vi "Main-Get and Set Height.vi"() -> ()   [LabVIEW 2014]
uses:
  Main-Stage-Based/(Global) Current handle and LaserPower_YCC.vi
  <vilib>/DAQmx/create/channels.llb/DAQmx Create Channel (AI-Voltage-Basic).vi
  <vilib>/DAQmx/configure/timing.llb/DAQmx Timing (Sample Clock).vi
  <vilib>/DAQmx/read.llb/DAQmx Read (Analog 1D DBL 1Chan NSamp).vi
panel:
  out "Surface position (um)":dbl
  out "Stage Array Shift (nm)":dbl
  in  "Change power?":bool
  in  "Set power (mV)":dbl=1000.0
  in  "Filter type 2":T1(ring)=enum."Moving-window avg"
  out "step size (nm)":dbl
  out "inital Laser power":dbl
  out "Avg to Hz":dbl
  out "Expect - Real move (nm)\nStage Offset\n+=more move\n-=less move":dbl
  in  "Tab Control":enum32{"Raw QPDz-Stage", "Filtered QPDz-Stage"}(tab)
  out "Raw XY Graph":T2(graph)
  out "Filtered XY Graph":T2(graph)
  in  "Set Height":bool
  in  "Set Height (nm)":dbl=300.0
  out "True rate?":bool
  in  "Avg points":i32=500
  out "traveling time (s)":dbl
  in  "Sampling Rate":dbl=32000.0 format="%0.2f"
  out "Position after move up":dbl
  in  "1/2 range  (um)":dbl=0.7000000000000001 format="%.3f"
  in  "scan rate  (um/s)":dbl=0.7 format="%.3f"
  out "Real Current Commanded position (um)":dbl=48.46734101118563 format="%0.5f"
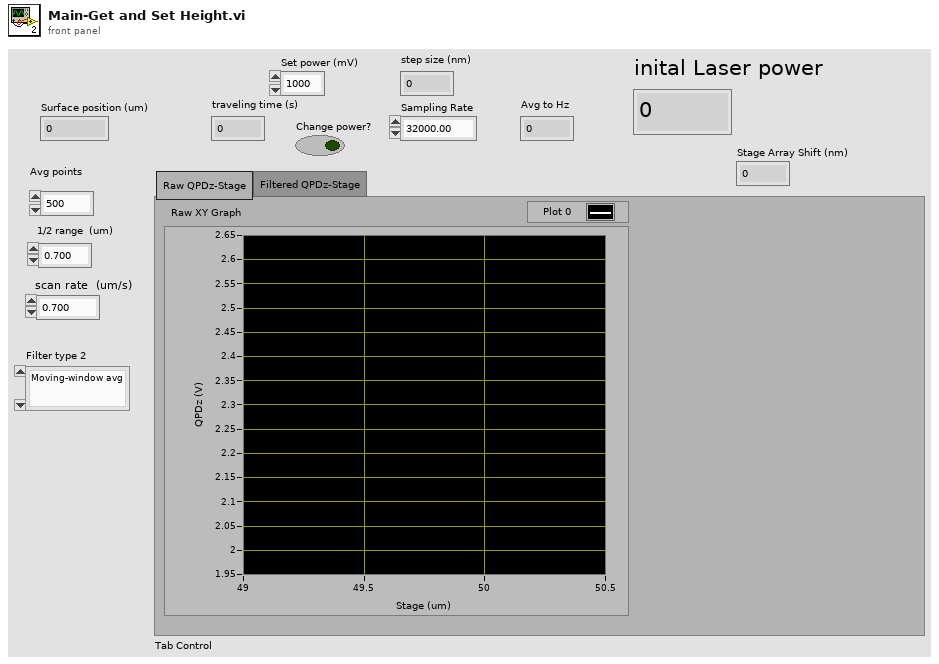
[diagram p1: front panel]
types:
  T1 = enum16{"Fixed-window avg", "Moving-window avg", "F+S-window avg", "S-G filter", "Fixed-window Median", "Moving-window Median "}
  T2 = cluster{"Filtered Stage Array":dbl[], "Filtered QPD data":dbl[]}
  T3 = cluster{"Correct Unfolded Stage Array (um)":dbl[], "Filtered QPD data":dbl[]}
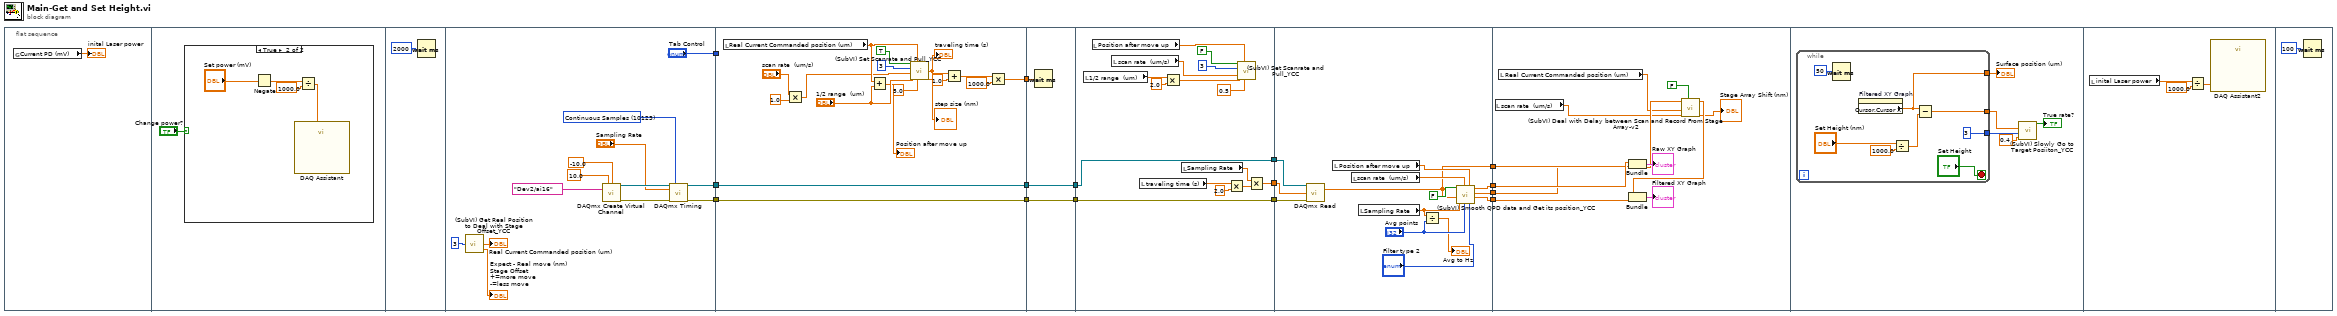
[diagram p0: block diagram]
diagram:
  n1 = flat-sequence {
    tunnel: [w26] -> w13
    tunnel: [w25] -> w9
    tunnel: ["Tab Control"] -> w1
    tunnel: [w46] -> w15
    tunnel: [w42] -> w14
    tunnel: w13 -> [w42]
    tunnel: [w41] -> w10
    tunnel: w9 -> [w41]
    tunnel: w1 -> [_]
    tunnel: w15 -> [w55]
    tunnel: w14 -> [w53]
    tunnel: [w54] -> w11
    tunnel: w10 -> [w54]
    tunnel: [w53] -> w7
    tunnel: [w66] -> w12
    tunnel: w11 -> [w66]
    tunnel: [w65] -> w8
    tunnel: w7 -> [w65]
    tunnel: [w63] -> w6
    tunnel: w12 -> [w84]
    tunnel: w8 -> [w83]
    tunnel: w6 -> [w82]
    tunnel: [w78] -> w5
    tunnel: [w77] -> w4
    tunnel: [w76] -> w3
    tunnel: [w75] -> w2
    tunnel: w5 -> [w90]
    tunnel: w4 -> [w95]
    tunnel: w3 -> [w94]
    tunnel: w2 -> [w93]
    frame #0 {
      n2 = global read "(Global) Current handle and LaserPower_YCC.vi" "Current PD (mV)"() -> (→"inital Laser power":dbl)
    }
    frame #1 {
      n3 = case shown="True" "Change power?" {
        frame False {
        }
        frame True {
          n4 = Negate(x="Set power (mV)") -> (-x=w20:dbl)
          n5 = Divide(x=w20, y=1000.0) -> (x/y=w18:dbl)
          n6 = call "DAQ Assistant"("data"=w18) -> ()  [unwired: 17 in, 2 out]
        }
      }
    }
    frame #2 {
      n7 = Wait (ms)(milliseconds to wait=u32 2000) -> ()  [unwired: 1 out]
    }
    frame #3 {
      w28 = 10123 items=["Finite Samples"=10178, "Continuous Samples"=10123, "Hardware Timed Single Point"=12522] ("sample mode")
      n8 = call "(SubVI) Get Real Position to Deal with Stage Offset_YCC.vi"("Axis"=3) -> ("Expect - Real move (nm)\nStage Offset\n+=more move\n-=less move"=→"Expect - Real move (nm)\nStage Offset\n+=more move\n-=less move":dbl, "Real Current Commanded position (um)"=→"Real Current Commanded position (um)":dbl)  [unwired: 3 in]
      n9 = call-poly <vilib>:"DAQmx Create Virtual Channel.vi"("maximum value"=10.0, "minimum value"=-10.0, "physical channels"=tag "Dev2/ai16") -> ("task out"=w29:refnum<k21>, "error out"=w30:errorcluster)  [unwired: 11 in]
      n10 = call-poly <vilib>:"DAQmx Timing.vi"("task/channels in"=w29, "sample mode"=w28, "rate"="Sampling Rate", "error in"=w30) -> ("task out"=w26:refnum<k21>, "error out"=w25:errorcluster)  [unwired: 10 in]
    }
    frame #4 {
      n11 = local read "Real Current Commanded position (um)"() -> (w45:dbl)
      n12 = Multiply(x="scan rate  (um/s)", y=1.0) -> (x*y=w36:dbl)
      n13 = Add(x=w45, y="1/2 range  (um)") -> (x+y=→"Position after move up":dbl)
      n14 = call "(SubVI) Set Scanrate and Pull_YCC.vi"("toward+ ?\nT=+, F=-"=TRUE ("toward+ ?\nT=+, F=-"), "Start From  (um)"=w45, "axis"=u32 3, "scan rate  (um/s)"=w36, "waiting time per point (ms)\nrange from 5ms to 0.167 ms"=5.0 ("waiting time per point (ms)\nrange from 5ms to 0.167 ms"), "range  (um)"="1/2 range  (um)") -> ("traveling time (s)"=w40:dbl, "step size (nm)"=→"step size (nm)":dbl)  [unwired: 1 out]
      "traveling time (s)" <- w40
      n15 = Add(x=w40, y=1.0) -> (x+y=w48:dbl)
      n16 = Multiply(x=w48, y=1000.0) -> (x*y=w46:dbl)
    }
    frame #5 {
      n17 = Wait (ms)(milliseconds to wait=w55) -> ()  [unwired: 1 out]
    }
    frame #6 {
      n18 = local read "1/2 range  (um)"() -> (w61:dbl)
      n19 = local read "Position after move up"() -> (w62:dbl)
      n20 = local read "scan rate  (um/s)"() -> (w68:dbl)
      n21 = local read "traveling time (s)"() -> (w57:dbl)
      n22 = Multiply(x=w61, y=2.0) -> (x*y=w59:dbl)
      n23 = local read "Sampling Rate"() -> (w64:dbl)
      n24 = Multiply(x=w57, y=2.0) -> (x*y=w56:dbl)
      n25 = call "(SubVI) Set Scanrate and Pull_YCC.vi"("toward+ ?\nT=+, F=-"=FALSE ("toward+ ?\nT=+, F=-"), "Start From  (um)"=w62, "axis"=u32 3, "scan rate  (um/s)"=w68, "waiting time per point (ms)\nrange from 5ms to 0.167 ms"=0.5 ("waiting time per point (ms)\nrange from 5ms to 0.167 ms"), "range  (um)"=w59) -> ()  [unwired: 3 out]
      n26 = Multiply(x=w64, y=w56) -> (x*y=w63:dbl)
    }
    frame #7 {
      n27 = call-poly <vilib>:"DAQmx Read.vi"("task/channels in"=w83, "number of samples per channel"=w82, "error in"=w84) -> ("data"=w75:dbl[])  [unwired: 10 in, 2 out]
      n28 = local read "Position after move up"() -> (w81:dbl)
      n29 = local read "scan rate  (um/s)"() -> (w80:dbl)
      n30 = local read "Sampling Rate"() -> (w74:dbl)
      n31 = Divide(x=w74, y="Avg points") -> (x/y=→"Avg to Hz":dbl)
      n32 = call "(SubVI) Smooth QPD data and Get its position_YCC.vi"("Filter type"="Filter type 2", "Initial position (um)"=w81, "Avg points"="Avg points", "scan rate  (um/s)"=w80, "Sampling rate (Hz)"=w74, "QPD data"=w75, "Direction\nT=+ \nF=-"=FALSE ("T=+ first\nF=- first")) -> ("Filtered QPD data"=w77:dbl[], "Filtered Stage Array"=w78:dbl[], "Raw Stage Array"=w76:dbl[])  [unwired: 2 in]
    }
    frame #8 {
      n33 = local read "scan rate  (um/s)"() -> (w87:dbl)
      n34 = local read "Real Current Commanded position (um)"() -> (w88:dbl)
      n35 = Bundle("Raw Stage Array"=w94, "data"=w93) -> (→"Raw XY Graph":cluster{"Raw Stage Array":dbl[], "data":dbl[]})  [unwired: 1 in]
      n36 = call "(SubVI) Deal with Delay between Scan and Record From Stage Array-v2.vi"("Toward first ?\nT=+, F=-"=FALSE ("Toward first ?\nT=+, F=-"), "Record scan rate  (um/s)"=w87, "Real initial position (um)"=w88, "Unfolded Stage Array (um)"=w90) -> ("Stage Array Shift (nm)"=→"Stage Array Shift (nm)":dbl, "Correct Unfolded Stage Array (um)"=w86:dbl[])  [unwired: 3 in, 1 out]
      n37 = Bundle("Correct Unfolded Stage Array (um)"=w86, "Filtered QPD data"=w95) -> (→"Filtered XY Graph":T3)  [unwired: 1 in]
    }
    frame #9 {
      n38 = while {
        tunnel: [w102] -> w99
        tunnel: [u32 3 ("axis")] -> w100
        tunnel: [w101] -> w96
        stop <- "Set Height" stop-if-true
        n39 = Wait (ms)(milliseconds to wait=u32 50) -> ()  [unwired: 1 out]
        n40 = property on="Filtered XY Graph" class="XYGraph (strict)"() -> ("Cursor.Cursor X"=w101:dbl)  [unwired: 2 in, 2 out]
        n41 = Divide(x="Set Height (nm)", y=1000.0) -> (x/y=w103:dbl)
        n42 = Subtract(x=w101, y=w103) -> (x-y=w102:dbl)
      }
      "Surface position (um)" <- w96
      n43 = call "(SubVI) Slowly Go to Target Posiiton_YCC.vi"("scan rate  (um/s)"=0.4, "axis"=w100, "Target position (um)"=w99) -> ("True rate?"=→"True rate?":bool)  [unwired: 1 in, 3 out]
    }
    frame #10 {
      n44 = local read "inital Laser power"() -> (w111:dbl)
      n45 = Divide(x=w111, y=1000.0) -> (x/y=w109:dbl)
      n46 = call "DAQ Assistant2"("data"=w109) -> ()  [unwired: 17 in, 2 out]
    }
    frame #11 {
      n47 = Wait (ms)(milliseconds to wait=u32 100) -> ()  [unwired: 1 out]
    }
  }
